vi "sub_update_cell.vi"(8 "error in (no error)":errorcluster, 9 "state":T1, 11 "Array In":bool[][](array[boolean])) -> (0 "error out":errorcluster, 3 "Array Out":bool[][](array[boolean]))   [LabVIEW 2018]
uses:
  index.ctl
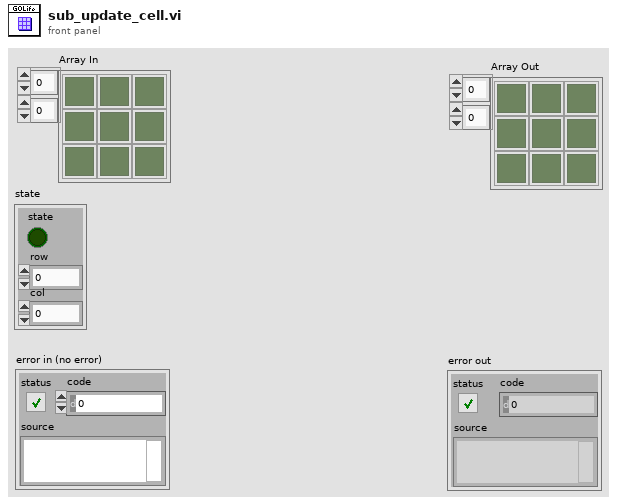
[diagram p1: front panel]
types:
  T1 = typedef "index.ctl" = cluster{"row":i32, "col":i32, "state":bool}
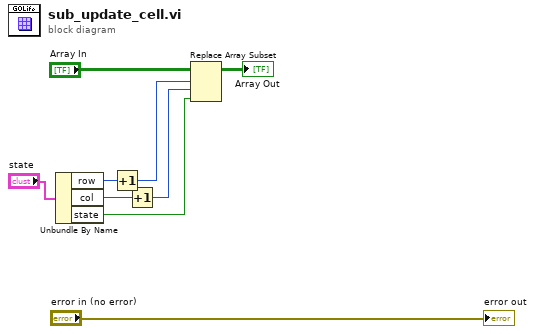
[diagram p0: block diagram]
diagram:
  n1 = Unbundle By Name("state") -> ("row"=w7:i32, "col"=w6:i32, "state"=w5:bool)
  n2 = Increment(x=w7) -> (x+1=w4:i32)
  n3 = Increment(x=w6) -> (x+1=w3:i32)
  n4 = Replace Array Subset(array="Array In", new element=w5, index (row)=w4, index (col)=w3) -> (→"Array Out":bool[][])
  "error out" <- "error in (no error)"
